vi "Write Min frequency.vi"(8 "error in (no error)":errorcluster, 10 "Min frequency":dbl, 11 "FEA_Model in":refnum<class "FEA_Model.lvclass">) -> (0 "error out":errorcluster, 3 "FEA_Model out":refnum<class "FEA_Model.lvclass">)   [LabVIEW 2021, in "FEA_Model.lvclass"]
uses:
  FEA_Model.lvclass
  FEA_Model.lvclass/FEA_Model.ctl
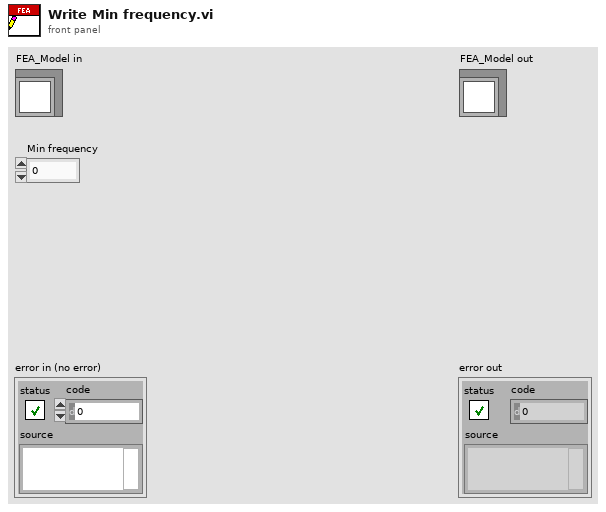
[diagram p1: front panel]
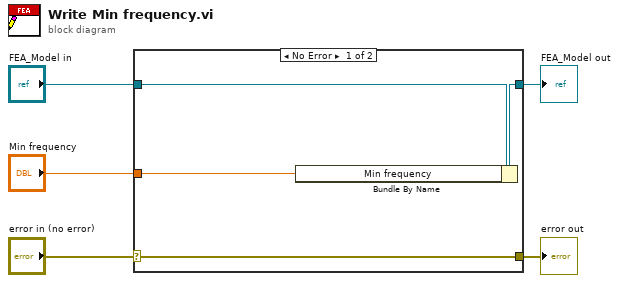
[diagram p0: block diagram]
diagram:
  n1 = case shown="No Error" "error in (no error)" {
    selector: "error in (no error)" -> [w9 w10]
    tunnel: [w9 w10] -> w4
    tunnel: [w7 w11] -> w2
    tunnel: "FEA_Model in" -> [w8 w11]
    tunnel: "Min frequency" -> [w6 _]
    frame No Error {
      n2 = Bundle By Name(cluster=w8, "Min frequency"=w6) -> (w7:refnum<class "FEA_Model.lvclass">)
    }
    frame Error {
    }
  }
  "error out" <- w4
  "FEA_Model out" <- w2
